vi "PZTManual.vi"(8 "error in (no error)":errorcluster, 11 "Cluster":T1 {"Z" max=50000 step=1; "Y" max=70000 step=1; "X" max=70000 step=1}) -> (0 "error out":errorcluster, 3 "Cluster 2":T1 caption="Cluster" {"Z" max=50000 step=1; "Y" max=70000 step=1; "X" max=70000 step=1})   [LabVIEW 2016]
panel:
  # "PZT Move"
  # "Step"
  # "Run"
  # "Step"
  # "Run"
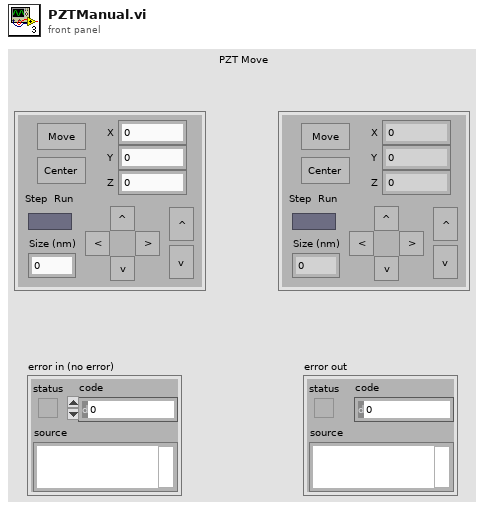
[diagram p1: front panel]
types:
  T1 = cluster{"Step/Run":bool, "Size (nm)":u32, "X-":bool, "X+":bool, "Y+":bool, "Y-":bool, "Z+":bool, "Z-":bool, "Center":bool, "Move":bool, "Z":u32, "Y":u32, "X":u32}
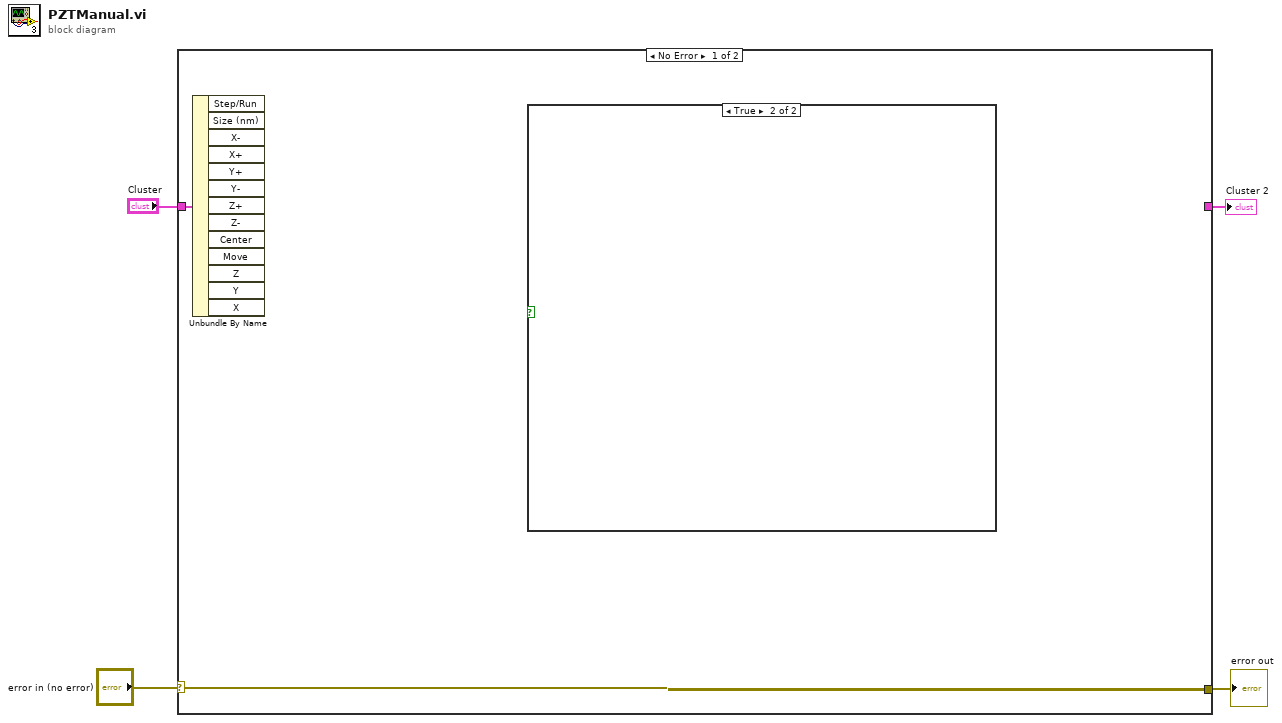
[diagram p0: block diagram]
diagram:
  n1 = case shown="No Error" "error in (no error)" {
    selector: "error in (no error)" -> [w5 w8]
    tunnel: "Cluster" -> [w6 w7]
    tunnel: [w5 w8] -> w2
    tunnel: [_ w7] -> w1
    frame No Error {
      n2 = Unbundle By Name(w6) -> ()  [unwired: 13 out]
      n3 = case shown="True" {
        selector: _ -> [_ _]
        frame False {
        }
        frame True {
        }
      }
    }
    frame Error {
    }
  }
  "error out" <- w2
  "Cluster 2" <- w1
